vi "Get UI Ref.vi"(8 "error in (no error)":errorcluster, 11 "9350 in":refnum<class "9350.lvclass">) -> (0 "error out":errorcluster, 1 "Show SubPanel?":bool, 2 "VI Refnum":refnum<vi>, 3 "9350 out":refnum<class "9350.lvclass">)   [LabVIEW 2017, in "Modules.lvlib" / "9350.lvclass"]
uses:
  9350.lvclass
  9350_UI.vi
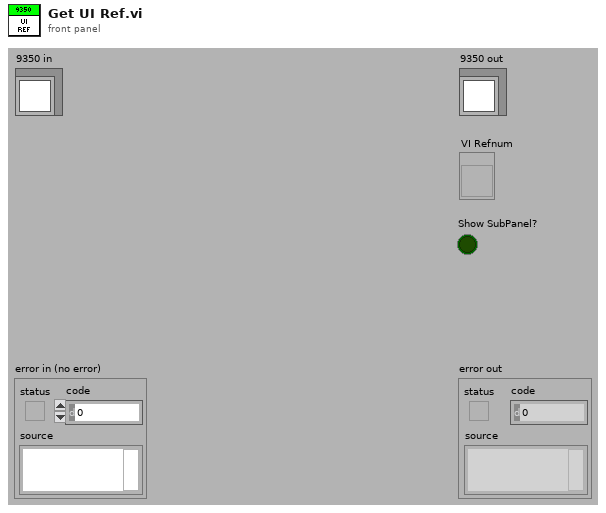
[diagram p1: front panel]
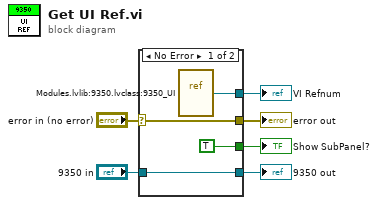
[diagram p0: block diagram]
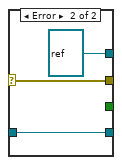
[diagram p2: hidden frame]
diagram:
  n1 = case shown="No Error" "error in (no error)" {
    selector: "error in (no error)" -> [w9 w13]
    tunnel: [w9 w13] -> w5
    tunnel: [w10 w12] -> w3
    tunnel: "9350 in" -> [w10 w12]
    tunnel: [TRUE _] -> w1
    tunnel: [w7 refnum<vi> refnum] -> w2
    frame No Error {
      n2 = vi-ref "Modules.lvlib:9350.lvclass:9350_UI.vi"() -> (w7:refnum<vi>)
    }
    frame Error {
    }
  }
  "error out" <- w5
  "9350 out" <- w3
  "VI Refnum" <- w2
  "Show SubPanel?" <- w1
